vi "sampled.vi"() -> ()   [LabVIEW 2020]
panel:
  out "x+y":dbl
  in  "x":dbl
  in  "y":dbl
  in  "stop":bool
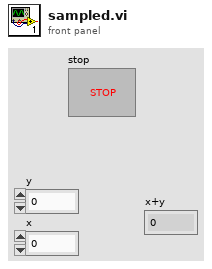
[diagram p1: front panel]
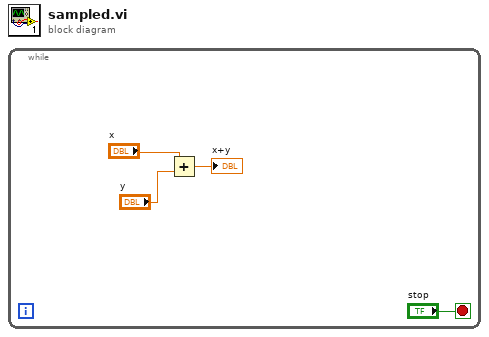
[diagram p0: block diagram]
diagram:
  n1 = while {
    stop <- "stop" stop-if-true
    n2 = Add(x="x", y="y") -> (x+y=→"x+y":dbl)
  }
